vi "setPosition_fw103.vi"(8 "waitTimeout":i32=500, 9 "Set position\n(deg) (float)":dbl, 11 "Method reference input":refnum<k24>) -> (1 "Current position (deg) (float)":i32 format="%.3f", 2 "error out":errorcluster, 3 "Method reference out":refnum<k24>)   [LabVIEW 2020]
uses:
  C:/Users/OPMuser/Documents/labview/fw103/Thorlabs.MotionControl.Benchtop.StepperMotorCLI.dll
  Thorlabs.MotionControl.Benchtop.StepperMotorCLI.dll
  <vilib>/Utility/error.llb/Error Cluster From Error Code.vi
  <vilib>/ErrorRing/Error Ring.xnode
panel:
  # "Move filter wheel VI"
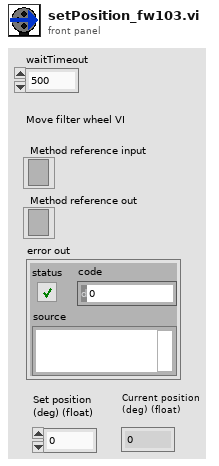
[diagram p1: front panel]
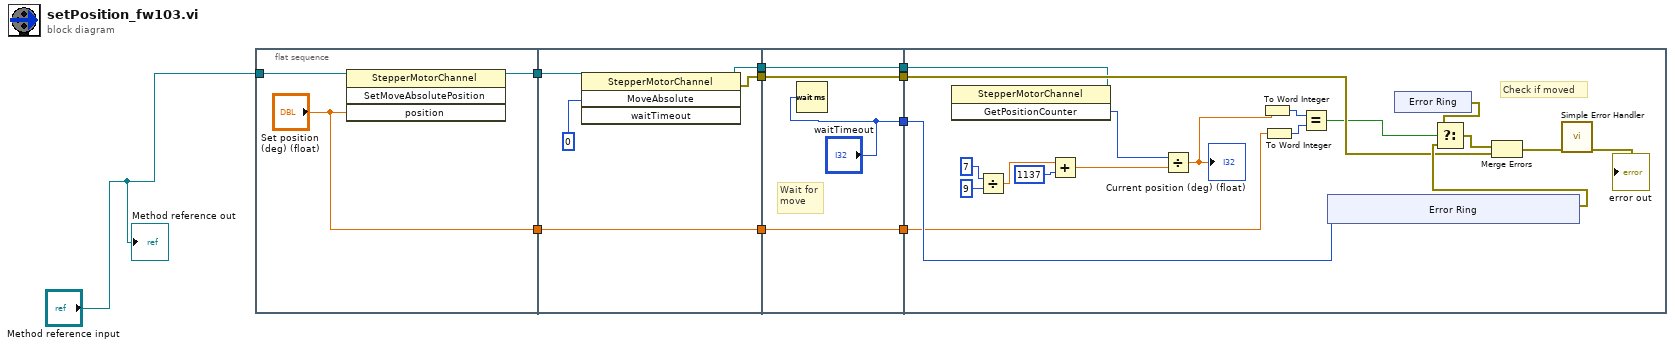
[diagram p0: block diagram]
diagram:
  n1 = flat-sequence {
    tunnel: [w13] -> w7
    tunnel: ["Set position\n(deg) (float)"] -> w2
    tunnel: "Method reference input" -> [w11]
    tunnel: [w17] -> w10
    tunnel: w7 -> [w16]
    tunnel: [w15] -> w5
    tunnel: [w14] -> w3
    tunnel: w2 -> [w14]
    tunnel: ["waitTimeout"] -> w9
    tunnel: [w22] -> w8
    tunnel: w10 -> [w22]
    tunnel: [w21] -> w6
    tunnel: w5 -> [w21]
    tunnel: [w20] -> w4
    tunnel: w3 -> [w20]
    tunnel: w9 -> [w40]
    tunnel: w8 -> [w36]
    tunnel: w6 -> [w34]
    tunnel: w4 -> [w26]
    frame #0 {
      n2 = invoke class="StepperMotorChannel" method="SetMoveAbsolutePosition"(reference=w11, "position"="Set position\n(deg) (float)") -> (reference out=w13:refnum<k24>)  [unwired: 2 in, 3 out]
    }
    frame #1 {
      n3 = invoke class="StepperMotorChannel" method="MoveAbsolute"(reference=w16, "waitTimeout"=0) -> (reference out=w15:refnum<k24>, error out=w17:errorcluster)  [unwired: 2 in, 2 out]
    }
    frame #2 {
      # "Wait for\nmove"
      n4 = Wait (ms)(milliseconds to wait="waitTimeout") -> ()  [unwired: 1 out]
    }
    frame #3 {
      # "Check if moved"
      n5 = invoke class="StepperMotorChannel" method="GetPositionCounter"(reference=w34) -> ("GetPositionCounter"=w28:i32)  [unwired: 2 in, 2 out]
      n6 = Divide(x=7, y=9) -> (x/y=w31:dbl)
      n7 = Add(x=w31, y=1137) -> (x+y=w29:dbl)
      n8 = Divide(x=w28, y=w29) -> (x/y=w27:dbl)
      "Current position (deg) (float)" <- w27
      n9 = To Word Integer(number=w27) -> (16bit integer=w25:i16)
      n10 = To Word Integer(number=w26) -> (16bit integer=w24:i16)
      n11 = Equal?(x=w25, y=w24) -> (x = y?=w23:bool)
      n12 = xnode "Error Ring"("parameter 0"=w40) -> ("error out"=w38:errorcluster)
      n13 = xnode "Error Ring"() -> ("error out"=w39:errorcluster)
      n14 = Select(t=w39, s=w23, f=w38) -> (s? t:f=w37:errorcluster)
      n15 = Merge Errors(w37, w36) -> (w35:errorcluster)
      "error out" <- w35
      n16 = call <vilib>:"Simple Error Handler.vi"("error in (no error)"=w35) -> ()  [unwired: 4 in, 5 out]
    }
  }
  "Method reference out" <- "Method reference input"
